vi "KEB Acceler to Trampa.vi"(10 "acc [1\\s^2] in":dbl, 11 "rpm max in":dbl) -> (3 "upper limit":dbl)   [LabVIEW 2019]
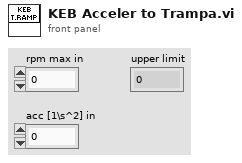
[diagram p1: front panel]
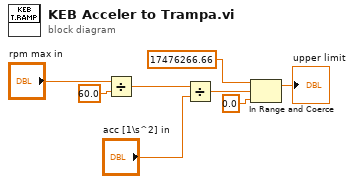
[diagram p0: block diagram]
diagram:
  n1 = Divide(x="rpm max in", y=60.0) -> (x/y=w4:dbl)
  n2 = Divide(x=w4, y="acc [1\\s^2] in") -> (x/y=w3:dbl)
  n3 = In Range and Coerce(upper limit=17476266.66, x=w3, lower limit=0.0) -> (coerced(x)=→"upper limit":dbl)  [unwired: 1 out]
